vi "subvi 2.vi"(8 "error in (no error)":errorcluster) -> (0 "error out":errorcluster)   [LabVIEW 2022 SP3]
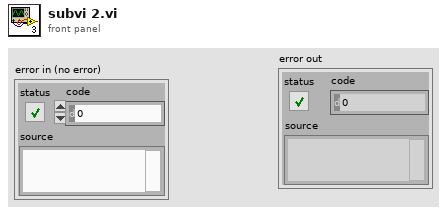
[diagram p1: front panel]
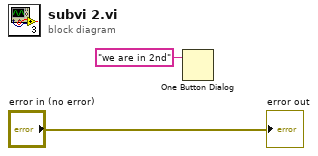
[diagram p0: block diagram]
diagram:
  n1 = One Button Dialog(message="we are in 2nd") -> ()  [unwired: 1 in, 1 out]
  "error out" <- "error in (no error)"
